vi "Read Channel Data.vi"(8 "error in (no error)":errorcluster, 11 "Adc Convertor in":refnum<class "Adc Convertor.lvclass">) -> (0 "error out":errorcluster, 2 "Channel Data":T1, 3 "Adc Convertor out":refnum<class "Adc Convertor.lvclass">)   [LabVIEW 2021, in "Adc Convertor.lvclass"]
uses:
  Adc Convertor.lvclass
  Controls/Channel Data.ctl
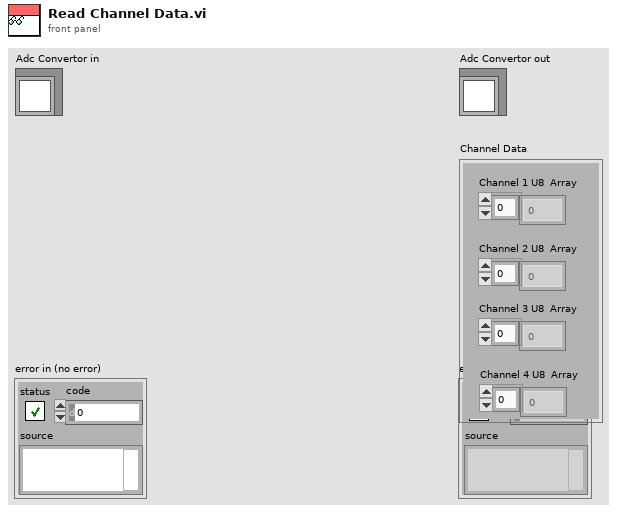
[diagram p1: front panel]
types:
  T1 = typedef "Channel Data.ctl" = cluster{"Channel 1 U8  Array":u8[], "Channel 2 U8  Array ":u8[], "Channel 3 U8  Array":u8[], "Channel 4 U8  Array":u8[]}
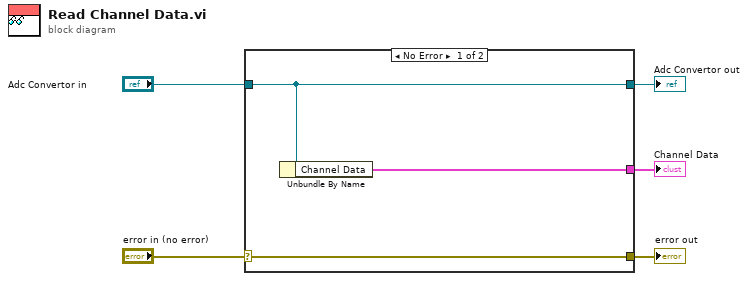
[diagram p0: block diagram]
diagram:
  n1 = case shown="No Error" "error in (no error)" {
    selector: "error in (no error)" -> [w8 w9]
    tunnel: [w8 w9] -> w4
    tunnel: [w7 w10] -> w2
    tunnel: "Adc Convertor in" -> [w7 w10]
    tunnel: [w6 _] -> w1
    frame No Error {
      n2 = Unbundle By Name(w7) -> ("Channel Data"=w6:T1)
    }
    frame Error {
    }
  }
  "error out" <- w4
  "Adc Convertor out" <- w2
  "Channel Data" <- w1
